vi "Flatten.vi"(8 "error in (no error)":errorcluster, 10 "Pretty Print?":bool, 11 "JSON Array in":refnum<class "JSON Array.lvclass">) -> (0 "error out":errorcluster, 2 "<JSON>":string)   [LabVIEW 2020, in "Library Commun.lvlib" / "JSON Array.lvclass"]
doc: "Converts an <b>JSON array</b> into <b>String</b>. Use <b>Pretty Print?</b> to auto-indent and distribute the string over different lines.\n\nCopyright 2012 James David Powell, Shaun Rumbell and Ton Plomp\nMore information on http://lavag.org/topic/16217-cr-json-labview"
uses:
  JSON Array.lvclass
  JSON Array.lvclass/JSON Array.ctl
  JSON Value/JSON Value.lvclass
  support/JSON support.lvlib
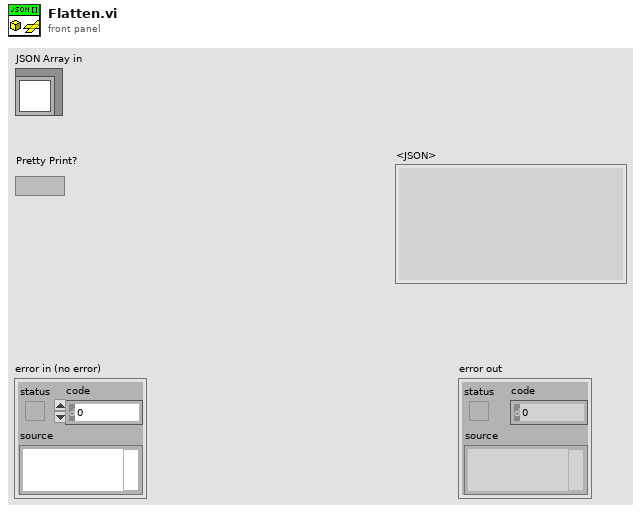
[diagram p1: front panel]
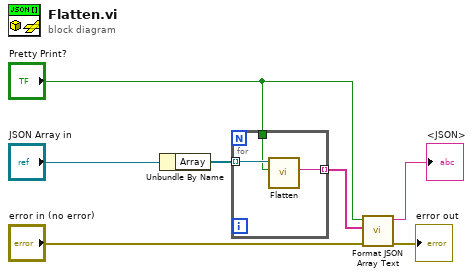
[diagram p0: block diagram]
diagram:
  n1 = Unbundle By Name("JSON Array in") -> ("Array"=w2:refnum<class "JSON Value.lvclass">[])
  n2 = for {
    tunnel: w2 -> [w10] mode=indexing
    tunnel: [w9] -> w3 mode=indexing
    tunnel: "Pretty Print?" -> [w8]
    n3 = call-dynamic "Flatten.vi"("Pretty Print?"=w8, "JSON Value in"=w10) -> ("<JSON>"=w9:string)  [unwired: 8 in, 1 out]
  }
  n4 = call "Format JSON Array Text.vi"("error in (no error)"="error in (no error)", "Array of JSON Text"=w3, "Pretty Print?"="Pretty Print?") -> ("error out"=→"error out":errorcluster, "<JSON>"=→"<JSON>":string)  [unwired: 7 in]
